vi "ALTS-2015 Status Log Module.vi"(7 "Options":enum16{"Init", "Write", "Close"}(ring), 8 "error in":errorcluster, 11 "Text to  Log":string) -> (0 "error out":errorcluster)   [LabVIEW 2013]
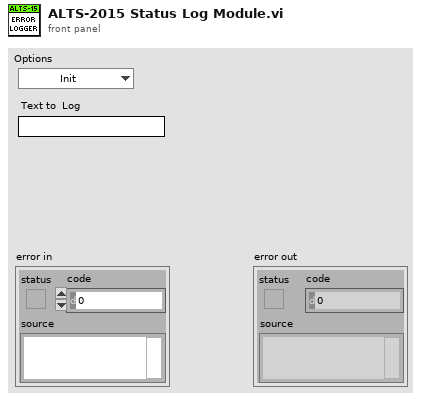
[diagram p1: front panel]
types:
  T1 = enum16{"open", "replace", "create", "open or create", "replace or create", "replace or create with confirmation"}
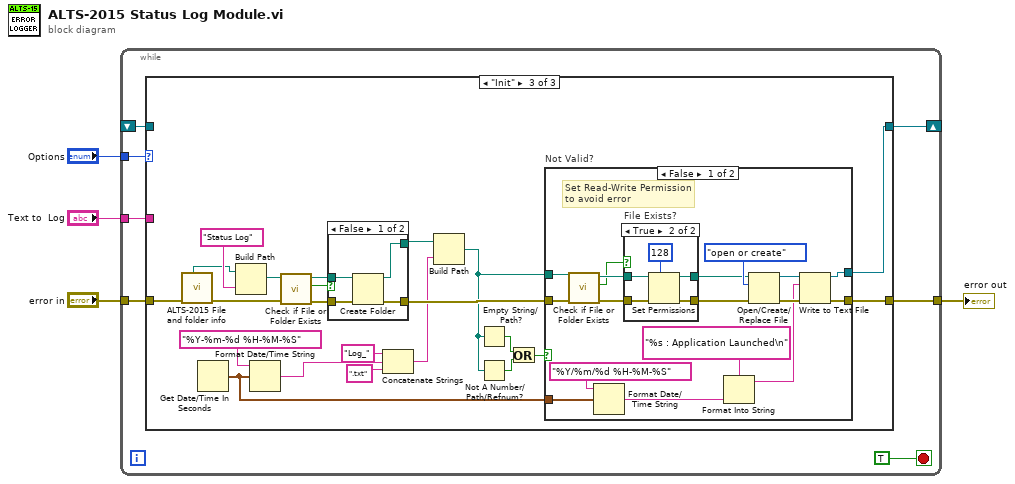
[diagram p0: block diagram]
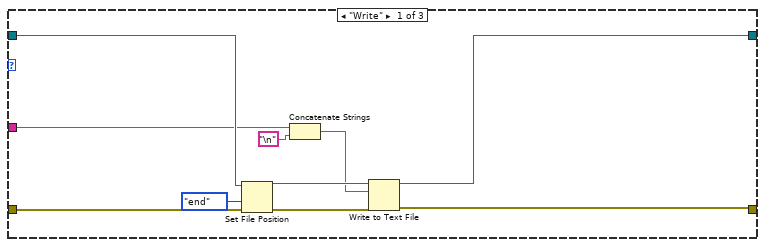
[diagram p2: hidden frame]
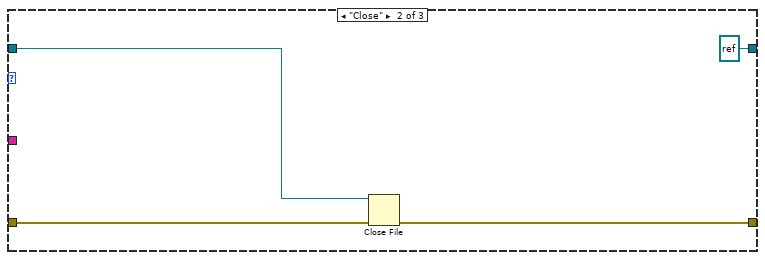
[diagram p3: hidden frame]
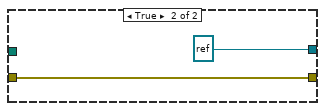
[diagram p5: hidden frame]
diagram:
  n1 = while {
    shift-right: [w11] -> _
    shift-left: _ -> [w9]
    tunnel: "Options" -> [w10]
    tunnel: "error in" -> [w8]
    tunnel: [w7] -> w2
    tunnel: "Text to  Log" -> [w6]
    stop <- TRUE stop-if-true
    n2 = case shown="\"Init\"" w10 {
      tunnel: [w15 refnum<file> refnum ("refnum out") w33] -> w11
      tunnel: w9 -> [w18 w24 _]
      tunnel: [w16 w25 w32] -> w7
      tunnel: w8 -> [w17 w22 w29]
      tunnel: w6 -> [w13 _ _]
      frame "Write" {
        n3 = Set File Position(refnum=w18, from (0:start)=enum16{"start", "end", "current"}."end", error in=w17) -> (refnum out=w21:refnum<file>, error out=w20:errorcluster)  [unwired: 1 out]
        n4 = Concatenate Strings(w13, "\n") -> (w12:string)
        n5 = Write to Text File(file (use dialog)=w21, text=w12, error in=w20) -> (refnum out=w15:refnum<file>, error out=w16:errorcluster)  [unwired: 2 out]
      }
      frame "Close" {
        n6 = Close File(refnum=w24, error in=w22) -> (error out=w25:errorcluster)  [unwired: 1 out]
      }
      frame "Init" {
        n7 = call "ALTS-2015 File and folder info.vi"("error in (no error)"=w29) -> ("error out"=w28:errorcluster, "Info Folder"=w30:path)  [unwired: 2 in, 7 out]
        n8 = Get Date/Time In Seconds() -> (seconds since 1Jan1904=w26:timestamp)
        n9 = Build Path(base path=w30, name or relative path="Status Log" ("string")) -> (appended path=w45:path)
        n10 = Format Date/Time String(time format string (%c)="%Y-%m-%d %H-%M-%S", seconds (now)=w26) -> (date/time string=w31:string)  [unwired: 1 out]
        n11 = call <vilib>:"Check if File or Folder Exists.vi"("error in (no error)"=w28, "path"=w45) -> ("error out"=w47:errorcluster, "file or folder exists?"=w39:bool, "dup path"=w46:path)  [unwired: 7 out]
        n12 = case shown="False" w39 {
          tunnel: w47 -> [w77 w78]
          tunnel: w46 -> [w76 w79]
          tunnel: [w75 w79] -> w43
          tunnel: [w74 w78] -> w42
          frame False {
            n13 = Create Folder(path (use dialog)=w76, error in=w77) -> (created path=w75:path, error out=w74:errorcluster)  [unwired: 2 out]
          }
          frame True {
          }
        }
        n14 = Concatenate Strings("Log_" ("string"), w31, ".txt" ("string")) -> (w34:string)
        n15 = Build Path(base path=w43, name or relative path=w34) -> (appended path=w36:path)
        n16 = Empty String/Path?(string/path=w36) -> (empty?=w37:bool)
        n17 = Not A Number/Path/Refnum?(number/path/refnum=w36) -> (NaN/Path/Refnum?=w38:bool)
        n18 = Or(x=w37, y=w38) -> (x .or. y?=w35:bool)
        n19 = case "Not Valid?" shown="False" w35 {
          tunnel: [w55 w72] -> w32
          tunnel: [w53 refnum<file> refnum ("refnum out")] -> w33
          tunnel: w42 -> [w59 w72]
          tunnel: w36 -> [w56 _]
          tunnel: w26 -> [w49 _]
          frame False {
            # "Set Read-Write Permission to avoid error"
            n20 = call <vilib>:"Check if File or Folder Exists.vi"("error in (no error)"=w59, "path"=w56) -> ("error out"=w58:errorcluster, "file or folder exists?"=w57:bool, "dup path"=w60:path)  [unwired: 7 out]
            n21 = Format Date/Time String(time format string (%c)="%Y/%m/%d %H-%M-%S", seconds (now)=w49) -> (date/time string=w48:string)  [unwired: 1 out]
            n22 = case "File Exists?" shown="True" w57 {
              tunnel: [w66 w70] -> w62
              tunnel: [w65 w69] -> w61
              tunnel: w60 -> [w66 w68]
              tunnel: w58 -> [w65 w67]
              frame False {
              }
              frame True {
                n23 = Set Permissions(7:i16 128 ("permissions"), 8:w67, 11:w68) -> (0:w69:errorcluster, 3:w70:path)  [unwired: 2 out]
              }
            }
            n24 = Format Into String(format string="%s : Application Launched\n", w48) -> (resulting string=w52:string)  [unwired: 2 in, 1 out]
            n25 = Open/Create/Replace File(file path (use dialog)=w62, error in=w61, operation (0:open)=T1."open or create") -> (refnum out=w54:refnum<file>, error out=w64:errorcluster)  [unwired: 3 in, 1 out]
            n26 = Write to Text File(file (use dialog)=w54, text=w52, error in=w64) -> (refnum out=w53:refnum<file>, error out=w55:errorcluster)  [unwired: 1 in, 1 out]
          }
          frame True {
          }
        }
      }
    }
  }
  "error out" <- w2
